vi "Patch_multipart_request.vi"   [LabVIEW 2016]
uses:
  Headers/Headers.ctl
  <vilib>/httpClient/MultipartData.ctl
  <vilib>/httpClient/LabVIEWHTTPClient.lvlib
types:
  T1 = typedef "LabVIEWHTTPClient.lvlib/MultipartData.ctl" = cluster{"Name":string, "Value":string, "File":path, "Filename":string, "MIME type":string}
  T2 = typedef "Headers.ctl" = cluster{"Name":string, "Value":string}[]
  T3 = typedef "URL_Data.ctl" = cluster{"Root":string, "Endpoint":string, "Request_URL":string}
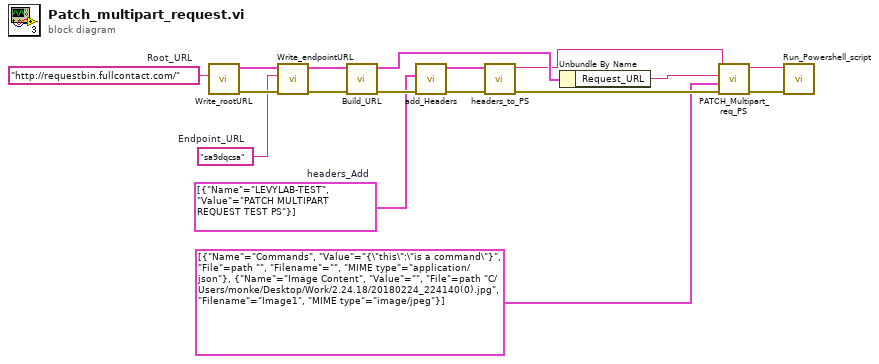
[diagram p0: block diagram]
diagram:
  w5 = T2 [{"Name"="LEVYLAB-TEST", "Value"="PATCH MULTIPART REQUEST TEST PS"}]  # headers_Add
  w7 = "sa9dqcsa"  # Endpoint_URL
  w8 = "http://requestbin.fullcontact.com/"  # Root_URL
  n1 = call "Write_rootURL.vi"("Root_URL"=w8) -> ("error out"=w9:errorcluster, "URL OUT"=w17:T3)  [unwired: 9 in]
  n2 = call "Write_endpointURL.vi"("error in"=w9, "Endpoint_URL"=w7, "URL IN"=w17) -> ("error out"=w10:errorcluster, "URL OUT"=w16:T3)  [unwired: 7 in]
  n3 = call "Build_URL.vi"("error in"=w10, "URL IN"=w16) -> ("error out"=w11:errorcluster, "URL OUT"=w15:T3)  [unwired: 8 in]
  n4 = call "add_Headers.vi"("error in"=w11, "headers_Add"=w5) -> ("error out"=w12:errorcluster, "Headers Out"=w6:T2)  [unwired: 8 in]
  n5 = call "headers_to_PS.vi"("error in"=w12, "Headers In"=w6) -> ("error out"=w13:errorcluster, "Headers_PS_Dict"=w2:string)  [unwired: 8 in]
  n6 = Unbundle By Name(w15) -> ("Request_URL"=w14:string)
  n7 = call "PATCH_Multipart_req_PS.vi"("error in"=w13, "Multipart Data In"=T1[] [{"Name"="Commands", "Value"="{\"this\":\"is a command\"}", "File"=path "", "Filename"="", "MIME type"="application/json"}, {"Name"="Image Content", "Value"="", "File"=path "C:/Users/monke/Desktop/Work/2.24.18/20180224_224140(0).jpg", "Filename"="Image1", "MIME type"="image/jpeg"}], 10:w14, "URL"=w2) -> ("error out"=w3:errorcluster, "Multipart PATCH Request"=w4:string)  [unwired: 6 in]
  n8 = call "Run_Powershell_script.vi"("error in"=w3, "Powershell Script"=w4) -> ()  [unwired: 7 in, 3 out]
